vi "Trim Flat Top.vi"(0 "Data In":dbl[](array[numeric])) -> (1 "Data Out (x,y)":cluster{i32[], dbl[]}, 2 "Trimmed Data (x,y)":cluster{i32[], dbl[]})   [LabVIEW 2012]
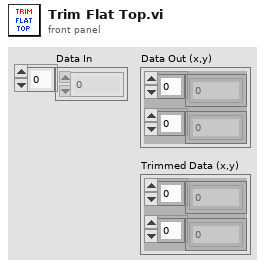
[diagram p1: front panel]
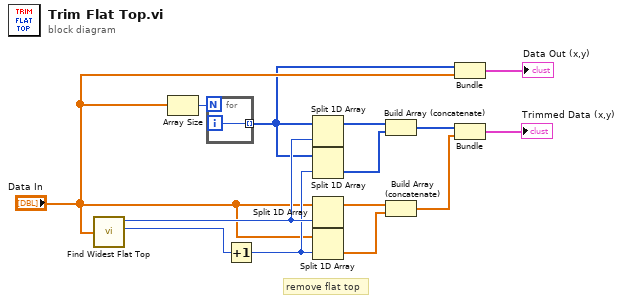
[diagram p0: block diagram]
diagram:
  # "remove flat top"
  n1 = call "Find Widest Flat Top.vi"("Data In"="Data In") -> ("start"=w8:i32, "end"=w13:i32)  [unwired: 2 out]
  n2 = Array Size(array="Data In") -> (size(s)=w11:i32)
  n3 = for {
    N: w11 -> [_]
    tunnel: [w15] -> w1 mode=indexing
    i -> [w15]
  }
  n4 = Increment(x=w13) -> (x+1=w7:i32)
  n5 = Split 1D Array(array=w1, index=w8) -> (first subarray=w10:i32[])  [unwired: 1 out]
  n6 = Split 1D Array(array=w1, index=w7) -> (second subarray=w9:i32[])  [unwired: 1 out]
  n7 = Split 1D Array(array="Data In", index=w8) -> (first subarray=w12:dbl[])  [unwired: 1 out]
  n8 = Split 1D Array(array="Data In", index=w7) -> (second subarray=w14:dbl[])  [unwired: 1 out]
  n9 = Build Array (concatenate)(w10, w9) -> (w3:i32[])
  n10 = Build Array (concatenate)(w12, w14) -> (w6:dbl[])
  n11 = Bundle(w1, "Data In"="Data In") -> (→"Data Out (x,y)":cluster{i32[], "Data In":dbl[]})  [unwired: 1 in]
  n12 = Bundle(w3, w6) -> (→"Trimmed Data (x,y)":cluster{i32[], dbl[]})  [unwired: 1 in]
